vi "rio_Global.vi"() -> ()   [LabVIEW 2015]
uses:
  <vilib>/Analysis/Matrix/Datatypes/RealMatrix.ctl
  <vilib>/Analysis/Matrix/NI_Matrix.lvlib
panel:
  out "time V":dbl
  out "C_timeyaw":dbl
  out "C_yaw_rate dt":dbl
  out "LCM_CON_T 2":T1={"hash"=6240213546654873975, "sys time"=0, "Auto"=FALSE, "Run"=FALSE, "Solenoid"=FALSE, "T lim"=FALSE, "brk_enc"=0, "B PWM"=0, "T PWM"=0, "ref_vel"=0.0, "ref_bkr_enc"=0.0, "ref_apv"=0.0, "ref_steer"=0.0, "net address"=0} {"net address" format="%08x"; "hash" format="%016x"}
  out "M_lane_right_old":dbl[](array[numeric])
  out "M_lane_left_old":dbl[](array[numeric])
  out "CON_INPUT_T 2":T2={"hash"=-1383086933477118758, "sys time"=0, "ref_vel"=0.0, "ref_steer"=0.0, "alert"=0} {"hash" format="%016x"}
  out "x_view 2":dbl[](array[numeric])=[0.0, 0.5, 1.0, 1.5, 2.0, 2.5, 3.0, 3.5, 4.0, 4.5, 5.0, 5.5, 6.0, 6.5, 7.0, 7.5, 8.0, 8.5, 9.0, 9.5, 10.0, 10.5, 11.0, 11.5, 12.0, 12.5, 13.0, 13.5, 14.0, 14.5, 15.0, 15.5, 16.0, 16.5, 17.0, 17.5, 18.0, 18.5, 19.0, 19.5, 20.0, 20.5, 21.0, 21.5, 22.0, 22.5, 23.0, 23.5, 24.0, 24.5, 25.0, 25.5, 26.0, 26.5, 27.0, 27.5, 28.0, 28.5, 29.0, 29.5, 30.0, 30.5, 31.0, 31.5, 32.0, 32.5, 33.0, 33.5, 34.0, 34.5, 35.0, 35.5, 36.0, 36.5, 37.0, 37.5, 38.0, 38.5, 39.0, 39.5, 40.0, 40.5, 41.0, 41.5, 42.0, 42.5, 43.0, 43.5, 44.0, 44.5, 45.0, 45.5, 46.0, 46.5, 47.0, 47.5, 48.0, 48.5, 49.0, 49.5, 50.0, 50.5, 51.0, 51.5, 52.0, 52.5, 53.0, 53.5, 54.0, 54.5, 55.0, 55.5, 56.0, 56.5, 57.0, 57.5, 58.0, 58.5, 59.0, 59.5, 60.0, 60.5, 61.0, 61.5, 62.0, 62.5, 63.0, 63.5, 64.0, 64.5, 65.0, 65.5, 66.0, 66.5, 67.0, 67.5, 68.0, 68.5, 69.0, 69.5, 70.0, 70.5, 71.0, 71.5, 72.0, 72.5, 73.0, 73.5, 74.0, 74.5, 75.0, 75.5, 76.0, 76.5, 77.0, 77.5, 78.0, 78.5, 79.0, 79.5, 80.0, 80.5, 81.0, 81.5, 82.0, 82.5, 83.0, 83.5, 84.0, 84.5, 85.0, 85.5, 86.0, 86.5, 87.0, 87.5, 88.0, 88.5, 89.0, 89.5, 90.0, 90.5, 91.0, 91.5, 92.0, 92.5, 93.0, 93.5, 94.0, 94.5, 95.0, 95.5, 96.0, 96.5, 97.0, 97.5, 98.0, 98.5, 99.0, 99.5, 100.0, 100.5, 101.0, 101.5, 102.0, 102.5, 103.0, 103.5, 104.0, 104.5, 105.0, 105.5, 106.0, 106.5, 107.0, 107.5, 108.0, 108.5, 109.0, 109.5, 110.0, 110.5, 111.0, 111.5, 112.0, 112.5, 113.0, 113.5, 114.0, 114.5, 115.0, 115.5, 116.0, 116.5, 117.0, 117.5, 118.0, 118.5, 119.0, 119.5, 120.0, 120.5, 121.0, 121.5, 122.0, 122.5, 123.0, 123.5, 124.0, 124.5, 125.0, 125.5, 126.0, 126.5, 127.0, 127.5, 128.0]
  out "Shift control":dbl
  out "LCM_CAN_RAW_SNAP":T3={"hash"=-8920902524919788889, "sys time"=0, "size"=0, "data"=[]} {"hash" format="%016x"}
  out "PWM Shift":dbl=1000.0 min=1000.0 max=2000.0 step=1.0
  out "steering angle":dbl min=1000.0 max=2000.0 step=1.0
  out "Const Brk FULL":dbl=80.0
  out "brake encoder":dbl
  out "C_time":u32
  out "T lim counter 2":u16
  out "T lim counter":u16
  out "T lim once":bool
  out "Throttle_Enable":bool
  out "T Lim":bool
  out "Ref_str_torque":dbl
  out "Ref_str_ang":dbl
  out "Ref_VS":dbl
  out "Car_name":string
  out "C_Brake":bool
  out "LCM_CAN_CAR_RAW_T":T4={"hash"=-386282380061490012, "sys time"=0, "car time"=0, "ID"=0, "data"=[]} {"hash" format="%016x"}
  out "LCM_CAN_EYE_RAW_T":T5={"hash"=-386282380061490012, "sys time"=0, "mobileye time"=0, "ID"=0, "data"=[]} {"hash" format="%016x"}
  out "time":dbl
  out "y_p 2":dbl[](array[numeric])
  out "x_p 2":dbl[](array[numeric])
  out "cmd steer":dbl=25.77230806 format="%#_12g"
  out "overall width":dbl=1.77546
  out "turn radius":dbl=5.50164
  out "wheel base":dbl=25.77230806 format="%#_12g"
  out "Auto SW":bool
  out "ratio":dbl=25.77230806 format="%#_12g"
  out "lane width":dbl
  out "y_p":dbl[](array[numeric])
  out "x_p":dbl[](array[numeric])
  out "x_view":dbl[](array[numeric])=[0.0, 0.5, 1.0, 1.5, 2.0, 2.5, 3.0, 3.5, 4.0, 4.5, 5.0, 5.5, 6.0, 6.5, 7.0, 7.5, 8.0, 8.5, 9.0, 9.5, 10.0, 10.5, 11.0, 11.5, 12.0, 12.5, 13.0, 13.5, 14.0, 14.5, 15.0, 15.5, 16.0, 16.5, 17.0, 17.5, 18.0, 18.5, 19.0, 19.5, 20.0, 20.5, 21.0, 21.5, 22.0, 22.5, 23.0, 23.5, 24.0, 24.5, 25.0, 25.5, 26.0, 26.5, 27.0, 27.5, 28.0, 28.5, 29.0, 29.5, 30.0, 30.5, 31.0, 31.5, 32.0, 32.5, 33.0, 33.5, 34.0, 34.5, 35.0, 35.5, 36.0, 36.5, 37.0, 37.5, 38.0, 38.5, 39.0, 39.5, 40.0, 40.5, 41.0, 41.5, 42.0, 42.5, 43.0, 43.5, 44.0, 44.5, 45.0, 45.5, 46.0, 46.5, 47.0, 47.5, 48.0, 48.5, 49.0, 49.5, 50.0, 50.5, 51.0, 51.5, 52.0, 52.5, 53.0, 53.5, 54.0, 54.5, 55.0, 55.5, 56.0, 56.5, 57.0, 57.5, 58.0, 58.5, 59.0, 59.5, 60.0, 60.5, 61.0, 61.5, 62.0, 62.5, 63.0, 63.5, 64.0, 64.5, 65.0, 65.5, 66.0, 66.5, 67.0, 67.5, 68.0, 68.5, 69.0, 69.5, 70.0, 70.5, 71.0, 71.5, 72.0, 72.5, 73.0, 73.5, 74.0, 74.5, 75.0, 75.5, 76.0, 76.5, 77.0, 77.5, 78.0, 78.5, 79.0, 79.5, 80.0, 80.5, 81.0, 81.5, 82.0, 82.5, 83.0, 83.5, 84.0, 84.5, 85.0, 85.5, 86.0, 86.5, 87.0, 87.5, 88.0, 88.5, 89.0, 89.5, 90.0, 90.5, 91.0, 91.5, 92.0, 92.5, 93.0, 93.5, 94.0, 94.5, 95.0, 95.5, 96.0, 96.5, 97.0, 97.5, 98.0, 98.5, 99.0, 99.5, 100.0, 100.5, 101.0, 101.5, 102.0, 102.5, 103.0, 103.5, 104.0, 104.5, 105.0, 105.5, 106.0, 106.5, 107.0, 107.5, 108.0, 108.5, 109.0, 109.5, 110.0, 110.5, 111.0, 111.5, 112.0, 112.5, 113.0, 113.5, 114.0, 114.5, 115.0, 115.5, 116.0, 116.5, 117.0, 117.5, 118.0, 118.5, 119.0, 119.5, 120.0, 120.5, 121.0, 121.5, 122.0, 122.5, 123.0, 123.5, 124.0, 124.5, 125.0, 125.5, 126.0, 126.5, 127.0, 127.5, 128.0]
  out "y_c":dbl[](array[numeric])
  out "x_c":dbl[](array[numeric])
  out "M_lane_center":dbl[](array[numeric])
  out "y_l":dbl[](array[numeric])
  out "x_l":dbl[](array[numeric])
  out "y_r":dbl[](array[numeric])
  out "x_r":dbl[](array[numeric])
  out "M_time":dbl
  out "C_mdps torque volt":dbl
  out "M_next lane right":dbl[][](array[numeric])
  out "M_next lane left":dbl[][](array[numeric])
  out "M_lane_right":dbl[](array[numeric])
  out "M_lane_left":dbl[](array[numeric])
  out "M_1sec":dbl[](array[numeric])
  out "steering torque":dbl min=1000.0 max=2000.0 step=1.0
  out "PWM Brake":dbl=1000.0 min=1000.0 max=2000.0 step=1.0
  out "PWM GAS":dbl=1000.0 min=1000.0 max=2000.0 step=1.0
  out "Solenoid":bool=TRUE
  out "M_vel_limit":dbl
  out "M_FCW":u8
  out "M_lane":dbl[](array[numeric])
  out "M_obs":dbl[][](array[numeric])
  out "M_STOP":bool
  out "M_headway":dbl
  out "C_Door":bool
  out "C_Right light":bool
  out "C_Left light":bool
  out "C_WHL_SPD_FL":dbl
  out "C_WHL_SPD_FR":dbl
  out "C_WHL_SPD_RL":dbl
  out "C_WHL_SPD_RR":dbl
  out "LCM PC":T6={"connection ID"=refnum, "net address"=0, "port"=7667}
  out "CON_INPUT_T":T7={"hash"=7122929053877479277, "sys time"=0, "ref_vel"=0.0, "ref_steer"=0.0} {"hash" format="%016x"}
  out "LCM_CON_T":T8={"hash"=4999688090526594712, "sys time"=0, "Auto"=FALSE, "Run"=FALSE, "Solenoid"=FALSE, "T lim"=FALSE, "brk_enc"=0, "B PWM"=0, "T PWM"=0, "ref_vel"=0.0, "ref_bkr_enc"=0.0, "ref_apv"=0.0, "ref_steer"=0.0} {"hash" format="%016x"}
  out "LCM_EYE_RAW_T":T9={"hash"=-8920902524919788889, "sys time"=0, "mobileye"=[]} {"hash" format="%016x"}
  out "LCM_POS_T":T10={"hash"=8611666821338907869, "sys time"=0, "dt"=0.0, "x"=0.0, "y"=0.0, "speed"=0.0, "heading"=0.0, "yaw_rate"=0.0} {"hash" format="%016x"}
  out "LCM_CAN_T":T11={"hash"=4925705798588944810, "sys time"=0, "time"=0.0, "yaw_rate"=0.0, "mdps torque"=0.0, "mdps str_ang"=0.0, "VS_CAN"=0.0, "lat_accel"=0.0, "mcp"=0.0, "accel pedal value"=0.0, "tps"=0.0, "odometer"=0.0, "battery voltage"=0.0, "WHL_SPD_RR"=0.0, "WHL_SPD_RL"=0.0, "WHL_SPD_FR"=0.0, "WHL_SPD_FL"=0.0} {"hash" format="%016x"}
  out "LCM":T6={"connection ID"=refnum, "net address"=0, "port"=7667}
  out "LCM_GGA_T":T12={"hash"=1114363806672425932, "sys time"=0, "time"=0.0, "x"=0.0, "y"=0.0, "h"=0.0, "numSV"=0, "postype"=0, "lag"=0, "hordev"=0.0, "lat"=0.0, "lon"=0.0, "hgt"=0.0, "map_idx"=0} {"hash" format="%016x"}
  out "LCM_RMC_T":T13={"hash"=2469426948741950939, "sys time"=0, "time"=0.0, "speed"=0.0, "heading"=0.0, "lat"=0.0, "lon"=0.0} {"hash" format="%016x"}
  out "K":T14=[[1.0, 0.0, 0.0], [0.0, 1.0, 0.0], [0.0, 0.0, 0.05], [0.0, 0.0, 0.0], [0.0, 0.0, 0.0]]
  out "Pp":T14=[[1.0, 0.0, 0.0, 0.0, 0.0], [0.0, 1.0, 0.0, 0.0, 0.0], [0.0, 0.0, 0.05, 0.0, 0.0], [0.0, 0.0, 0.0, 0.0188, 0.0], [0.0, 0.0, 0.0, 0.0, 0.0017]]
  out "H":T14=[[1.0, 0.0, 0.0, 0.0, 0.0], [0.0, 1.0, 0.0, 0.0, 0.0], [0.0, 0.0, 0.0, 1.0, 0.0]]
  out "R":T14=[[10.0, 0.0, 0.0], [0.0, 10.0, 0.0], [0.0, 0.0, 0.5]]
  out "Q":T14=[[0.5, 0.0, 0.0, 0.0, 0.0], [0.0, 0.5, 0.0, 0.0, 0.0], [0.0, 0.0, 0.1, 0.0, 0.0], [0.0, 0.0, 0.0, 0.0341, 0.0], [0.0, 0.0, 0.0, 0.0, 0.0017]]
  out "P":T14=[[1.0, 0.0, 0.0, 0.0, 0.0], [0.0, 1.0, 0.0, 0.0, 0.0], [0.0, 0.0, 0.1, 0.0, 0.0], [0.0, 0.0, 0.0, 0.0341, 0.0], [0.0, 0.0, 0.0, 0.0, 0.0017]]
  out "gps_pos 2":dbl[](array[numeric]) format="%#_19f"
  out "gps_vel 2":dbl[](array[numeric]) format="%#_19f"
  out "gps_pos 1":dbl[](array[numeric]) format="%#_19f"
  out "gps_vel 1":dbl[](array[numeric]) format="%#_19f"
  out "C_ts":dbl
  out "C_MCP":dbl
  out "Ref MCP":dbl
  out "Ref APV":dbl
  out "C_VS_CAN":dbl
  out "C_mdps str_ang":dbl
  out "C_mdps torque":dbl
  out "C_odometer":dbl
  out "C_gear selector disp":u8
  out "C_battery voltage":dbl
  out "C_APV":dbl
  out "C_tps":dbl
  out "C_lat_accel":dbl
  out "C_yaw_rate":dbl
  out "Auto":bool
  out "Run":bool
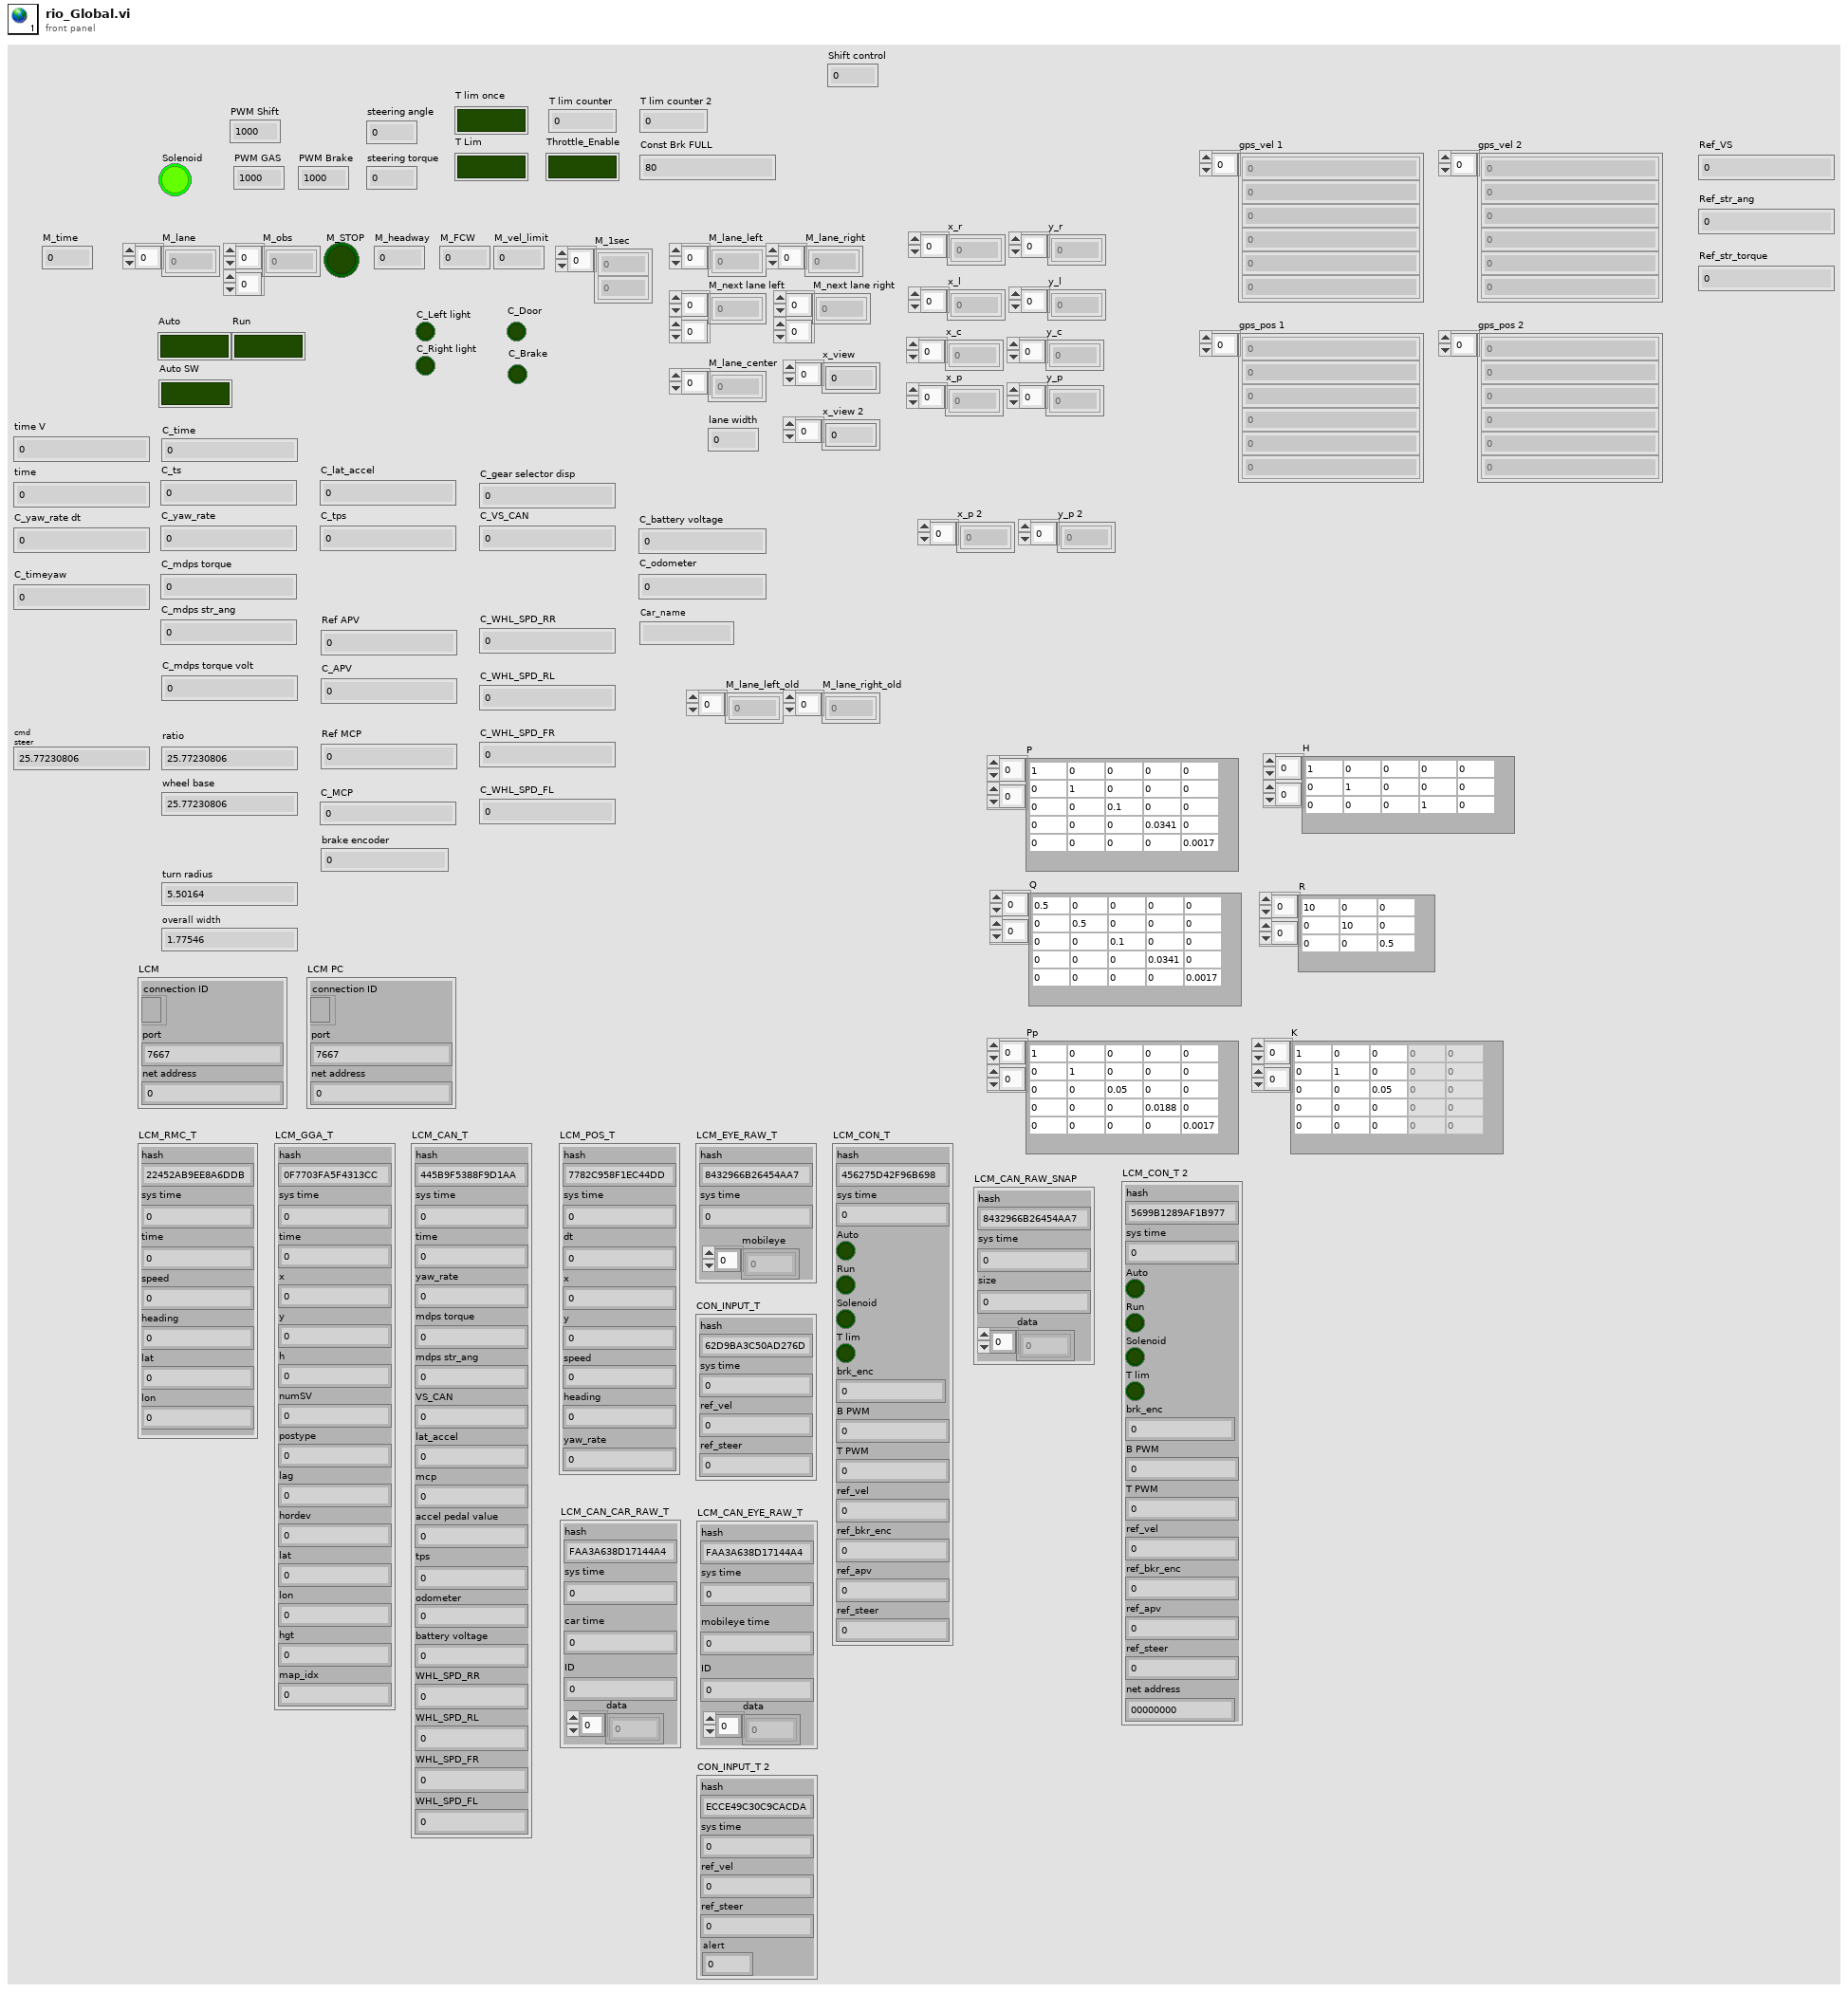
[diagram p1: front panel]
types:
  T1 = cluster{"hash":i64, "sys time":i64, "Auto":bool, "Run":bool, "Solenoid":bool, "T lim":bool, "brk_enc":u8, "B PWM":u16, "T PWM":u16, "ref_vel":dbl, "ref_bkr_enc":dbl, "ref_apv":dbl, "ref_steer":dbl, "net address":u32}
  T2 = cluster{"hash":i64, "sys time":i64, "ref_vel":dbl, "ref_steer":dbl, "alert":u8}
  T3 = cluster{"hash":i64, "sys time":i64, "size":i32, "data":u8[]}
  T4 = cluster{"hash":i64, "sys time":i64, "car time":u32, "ID":u32, "data":u8[]}
  T5 = cluster{"hash":i64, "sys time":i64, "mobileye time":u32, "ID":u32, "data":u8[]}
  T6 = cluster{"connection ID":refnum<k16>, "net address":u32, "port":u16}
  T7 = cluster{"hash":i64, "sys time":i64, "ref_vel":dbl, "ref_steer":dbl}
  T8 = cluster{"hash":i64, "sys time":i64, "Auto":bool, "Run":bool, "Solenoid":bool, "T lim":bool, "brk_enc":u8, "B PWM":u16, "T PWM":u16, "ref_vel":dbl, "ref_bkr_enc":dbl, "ref_apv":dbl, "ref_steer":dbl}
  T9 = cluster{"hash":i64, "sys time":i64, "mobileye":u8[]}
  T10 = cluster{"hash":i64, "sys time":i64, "dt":dbl, "x":dbl, "y":dbl, "speed":dbl, "heading":dbl, "yaw_rate":dbl}
  T11 = cluster{"hash":i64, "sys time":i64, "time":dbl, "yaw_rate":dbl, "mdps torque":dbl, "mdps str_ang":dbl, "VS_CAN":dbl, "lat_accel":dbl, "mcp":dbl, "accel pedal value":dbl, "tps":dbl, "odometer":dbl, "battery voltage":dbl, "WHL_SPD_RR":dbl, "WHL_SPD_RL":dbl, "WHL_SPD_FR":dbl, "WHL_SPD_FL":dbl}
  T12 = cluster{"hash":i64, "sys time":i64, "time":dbl, "x":dbl, "y":dbl, "h":dbl, "numSV":i32, "postype":i32, "lag":i32, "hordev":dbl, "lat":dbl, "lon":dbl, "hgt":dbl, "map_idx":i32}
  T13 = cluster{"hash":i64, "sys time":i64, "time":dbl, "speed":dbl, "heading":dbl, "lat":dbl, "lon":dbl}
  T14 = typedef "NI_Matrix.lvlib/RealMatrix.ctl" = dbl[][]
diagram:
